vi "UHR-Fleezers Control (host) - 12.1_Jonathan.vi"() -> ()   [LabVIEW 2012] (continued)
            n2498 = VISA Write(VISA resource name=w4134, write buffer=w4133) -> (VISA resource name out=w4130:refnum<visa-resource-name>)  [unwired: 1 in, 2 out]
            n2499 = Concatenate Strings("cvolume" ("string"), "\r") -> (w4131:string)
            n2500 = VISA Write(VISA resource name=w4130, write buffer=w4131) -> (VISA resource name out=w4125:refnum<visa-resource-name>)  [unwired: 1 in, 2 out]
            n2501 = Concatenate Strings("wrun" ("string"), "\r") -> (w4126:string)
            n2502 = VISA Write(VISA resource name=w4125, write buffer=w4126) -> ()  [unwired: 1 in, 3 out]
          }
        }
      }
      event "Flip Green Filter": Value Change {
        n2503 = event-data() -> ()  [unwired: 7 out]
        n2504 = Not(x="Flip Green Filter") -> (.not. x?=w4144:bool)
        n2505 = local write "Flip Green Filter"(w4144) -> ()
        n2506 = flat-sequence {
          tunnel: w4152 -> [w4157]
          tunnel: w4151 -> [w4156]
          tunnel: [w4154] -> w4149
          tunnel: [w4153] -> w4148
          tunnel: [w4159] -> w4147
          tunnel: w4149 -> [w4159]
          tunnel: [w4158] -> w4146
          tunnel: w4148 -> [w4158]
          tunnel: w4147 -> [w4163]
          tunnel: w4146 -> [w4162]
          tunnel: [w4161] -> w4150
          frame #0 {
            n2507 = xnode "Read/Write Control"("FPGA VI Reference In"=w4157, "error in"=w4156, "Green Filter Flipper"=TRUE) -> ("FPGA VI Reference Out"=w4154:T20, "error out"=w4153:errorcluster)
          }
          frame #1 {
            n2508 = Wait (ms)(milliseconds to wait=u32 100) -> ()  [unwired: 1 out]
          }
          frame #2 {
            n2509 = xnode "Read/Write Control"("FPGA VI Reference In"=w4163, "error in"=w4162, "Green Filter Flipper"=FALSE) -> ("error out"=w4161:errorcluster)  [unwired: 1 out]
          }
        }
      }
      event "Pump 1 contents", "Pump 3 contents": Value Change {
        n2510 = event-data() -> ()  [unwired: 7 out]
        n2511 = local read "Pump 1 contents"() -> (→"Pump 1 cont disp":string)
        n2512 = local read "Pump 3 contents"() -> (→"Pump 3 cont disp":string)
      }
      event "Reset Trap Pos. FB": Value Change {
        n2513 = event-data() -> ()  [unwired: 7 out]
        n2514 = xnode "Read/Write Control"("FPGA VI Reference In"=w4169, "error in"=w4168, "Trap Pos. FB Reset"="Reset Trap Pos. FB") -> ()  [unwired: 2 out]
      }
      event "Rem fb disp offset": Value Change {
        n2515 = event-data() -> ()  [unwired: 7 out]
        n2516 = local write "Rem fb disp offset"(FALSE ("Rem fb disp offset")) -> ()
        n2517 = local read "Mean T1 Position (nm)"() -> (w4171:dbl)
        n2518 = local read "FB Trap Pos Offset"() -> (w4172:dbl)
        n2519 = Subtract(x=w4172, y=w4171) -> (x-y=w4170:dbl)
        n2520 = local write "FB Trap Pos Offset"(w4170) -> ()
      }
      event "Threshold (nm)": Value Change {
        n2521 = event-data() -> ()  [unwired: 7 out]
        n2522 = flat-sequence {
          tunnel: w4176 -> [w4184]
          tunnel: w4175 -> [w4183]
          tunnel: [w4177] -> w4174
          tunnel: w4174 -> [w4190]
          frame #0 {
            n2523 = xnode "Read/Write Control"("FPGA VI Reference In"=w4184, "error in"=w4183) -> ("FPGA VI Reference Out"=w4180:T20, "error out"=w4179:errorcluster, "FPGA TTrig Thresh"=w4181:i64)
            n2524 = local read "Threshold stored (nm)"() -> (w4189:dbl)
            n2525 = local read "Threshold (nm)"() -> (w4177:dbl)
            n2526 = local read "AOM X Cal (nm/MHz)"() -> (w4187:dbl)
            n2527 = Subtract(x=w4177, y=w4189) -> (x-y=w4188:dbl)
            n2528 = Divide(x=w4188, y=w4187) -> (x/y=w4185:dbl)
            n2529 = call "IR AOM freq to word.vi"("Frequency In (MHz)"=w4185) -> ("Frequency Word Out (double)"=w4186:dbl)
            n2530 = To Quad Integer(1:w4186) -> (0:w4182:i64)
            n2531 = Add(x=w4181, y=w4182) -> (x+y=w4178:i64)
            n2532 = xnode "Read/Write Control"("FPGA VI Reference In"=w4180, "error in"=w4179, "FPGA TTrig Thresh"=w4178) -> ()  [unwired: 2 out]
          }
          frame #1 {
            "Threshold stored (nm)" <- w4190
          }
        }
      }
      event "FB Trig Integrate": Value Change {
        n2533 = event-data() -> ()  [unwired: 7 out]
        n2534 = local read "FB Trig Integrate"() -> (w4192:u32)
        n2535 = xnode "Read/Write Control"("FPGA VI Reference In"=w4194, "error in"=w4193, "FB Trig Integrate"=w4192) -> ("error out"=w4191:errorcluster)  [unwired: 1 out]
      }
      event "11": Value Change {
        n2536 = event-data() -> ()  [unwired: 7 out]
        n2537 = local read "11"() -> (w4195:bool)
        n2538 = case shown="True" w4195 {
          frame False {
          }
          frame True {
            n2539 = local read "Messages"() -> (w4197:string)
            n2540 = call "Update messages.vi"("Message to add"="You kicked it up to 11!", "Old message string"=w4197) -> ("New message string"=w4198:string)
            n2541 = call <vilib>:"Beep.vi"() -> ()  [unwired: 12 in]
            n2542 = local write "Messages"(w4198) -> ()
          }
        }
      }
      event "Trap Pos. FB ON": Value Change {
        n2543 = event-data() -> ()  [unwired: 7 out]
        n2544 = xnode "Read/Write Control"("FPGA VI Reference In"=w4201, "error in"=w4200, "Force feedback"="Trap Pos. FB ON") -> ()  [unwired: 2 out]
      }
      event "Remove Action Offset": Value Change {
        n2545 = event-data() -> ()  [unwired: 7 out]
        n2546 = local write "Remove Action Offset"(FALSE ("Remove Action Offset")) -> ()
        n2547 = local read "Trap Pos. FB Mult Factor"() -> (w4206:i64)
        n2548 = local read "Trap Pos FB Action"() -> (w4204:i64)
        n2549 = local read "Trap Pos. FB Offset Factor"() -> (w4202:i64)
        n2550 = Multiply(x=w4206, y=w4204) -> (x*y=w4205:i64)
        n2551 = Add(x=w4205, y=w4202) -> (x+y=w4203:i64)
        n2552 = local write "Trap Pos. FB Offset Factor"(w4203) -> ()
        n2553 = xnode "Read/Write Control"("FPGA VI Reference In"=w4209, "error in"=w4208, "Trap Pos. FB Offset Factor"=w4203) -> ()  [unwired: 2 out]
      }
      event "Remove Unwinding Offset": Value Change {
        n2554 = event-data() -> ()  [unwired: 7 out]
        n2555 = local write "Remove Unwinding Offset"(FALSE ("Remove Action Offset")) -> ()
        n2556 = local read "Trap Pos. FB Mult Factor"() -> (w4221:i64)
        n2557 = local read "Trap Pos FB Action"() -> (w4219:i64)
        n2558 = local read "Trap Pos. FB Offset Factor"() -> (w4218:i64)
        n2559 = Multiply(x=w4221, y=w4219) -> (x*y=w4220:i64)
        n2560 = local read "Trap Pos. FB Mult Factor"() -> (w4217:i64)
        n2561 = Add(x=w4220, y=w4218) -> (x+y=w4211:i64)
        n2562 = Multiply(x=32768, y="factor") -> (x*y=w4214:dbl)
        n2563 = Multiply(x=w4214, y=w4217) -> (x*y=w4216:dbl)
        n2564 = Subtract(x=w4211, y=w4216) -> (x-y=w4215:dbl)
        n2565 = To Quad Integer(1:w4215) -> (0:w4210:i64)
        n2566 = xnode "Read/Write Control"("FPGA VI Reference In"=w4224, "error in"=w4223, "Trap Pos. FB Offset Factor"=w4210) -> ()  [unwired: 2 out]
        n2567 = local write "Trap Pos. FB Offset Factor"(w4210) -> ()
      }
      event "Trap Pos. FB Range", "Trap Pos. FB Gains", "Trap Pos. FB Mult Factor", "Trap Pos. FB Offset Factor", "Trap Pos FB Negate Action", "Trap Pos FB Monitor\nT1 or T2", "Differential FB?", "Negate Diff?": Value Change {
        n2568 = event-data() -> ()  [unwired: 7 out]
        n2569 = local read "Negate Diff?"() -> (w4225:bool)
        n2570 = xnode "Read/Write Control"("FPGA VI Reference In"=w4235, "error in"=w4234, "Trap Pos. FB Range"="Trap Pos. FB Range", "Trap Pos. FB Gains"="Trap Pos. FB Gains", "Trap Pos. FB Mult Factor"="Trap Pos. FB Mult Factor", "Trap Pos. FB Offset Factor"="Trap Pos. FB Offset Factor", "Trap Pos FB Negate Action"="Trap Pos FB Negate Action", "Trap Pos FB Monitor T1 or T2"="Trap Pos FB Monitor\nT1 or T2", "AI1 X Scale"="Trap Pos. AI1 X Pre-scale", "Negate Diff?"=w4225, "Diff FB Measurement?"="Differential FB?") -> ()  [unwired: 2 out]
      }
      event "Trap Pos FB SP", "Trap Pos FB SP 2", "Use SP 2": Value Change {
        n2571 = event-data() -> ()  [unwired: 7 out]
        n2572 = Select(t="Trap Pos FB SP 2", s="Use SP 2", f="Trap Pos FB SP") -> (s? t:f=w4236:fxp<+/-,16,1>)
        n2573 = xnode "Read/Write Control"("FPGA VI Reference In"=w4241, "error in"=w4240, "Trap Pos. FB SP"=w4236) -> ()  [unwired: 2 out]
      }
      event "Offset SP2 from SP1": Value Change {
        n2574 = event-data() -> ()  [unwired: 7 out]
        n2575 = local read "Trap Pos FB SP"() -> (w4244:fxp<+/-,16,1>)
        n2576 = Add(x=w4244, y="SP2 Offset") -> (x+y=w4242:fxp<+/-,16,1>)
        n2577 = property on="Trap Pos FB SP 2" class="DigNum (strict)"("Val(Sgnl)"=w4242) -> ()  [unwired: 2 in, 2 out]
        n2578 = local write "Offset SP2 from SP1"(FALSE ("Offset SP2 from SP1")) -> ()
      }
      event "Set Reading to\nSetpoint": Value Change {
        # "This is the actual PID input signal"
        n2579 = event-data() -> ()  [unwired: 7 out]
        n2580 = local write "Set Reading to\nSetpoint"(FALSE ("Set SP to Reading")) -> ()
        n2581 = xnode "Read/Write Control"("FPGA VI Reference In"=w4250, "error in"=w4249) -> ("FPGA VI Reference Out"=w4248:T20, "error out"=w4247:errorcluster, "Trap Pos FB Int-Norm Signal"=w4246:fxp<+/-,16,1>)
        n2582 = local read "Differential FB?"() -> (w4251:bool)
        n2583 = case shown="False" w4251 {
          tunnel: [w4256 w4263] -> w4253
          tunnel: w4246 -> [w4254 w4263]
          frame False {
            n2584 = local read "Trap Pos FB Monitor\nT1 or T2"() -> (w4259:bool)
            n2585 = local read "Trap X AI1 (DMA)"() -> (w4262:T14)
            n2586 = Unbundle By Name(w4262) -> ("Set 1"=w4261:fxp<+/-,16,1>, "Set 2"=w4260:fxp<+/-,16,1>)
            n2587 = Select(t=w4261, s=w4259, f=w4260) -> (s? t:f=w4258:fxp<+/-,16,1>)
            n2588 = Not(x="Set SP Using...") -> (.not. x?=w4255:bool)
            n2589 = Select(t=w4254, s=w4255, f=w4258) -> (s? t:f=w4256:fxp<+/-,16,1>)
          }
          frame True {
          }
        }
        n2590 = xnode "Read/Write Control"("FPGA VI Reference In"=w4248, "error in"=w4247, "Trap Pos. FB SP"=w4253) -> ()  [unwired: 2 out]
        n2591 = local write "Trap Pos FB SP"(w4253) -> ()
      }
      event "Trap Pos. FB Out Scale 2^n": Value Change {
        n2592 = event-data() -> ()  [unwired: 7 out]
        n2593 = Scale By Power Of 2(n="Trap Pos. FB Out Scale 2^n", x=ext 1.0) -> (x*2^n=w4264:ext)
        n2594 = property on="Trap Pos. FB Mult Factor" class="DigNum (strict)"("Val(Sgnl)"=w4264) -> ()  [unwired: 2 in, 2 out]
      }
      event "Trap Pos FB Int Count": Value Change {
        n2595 = event-data() -> ()  [unwired: 7 out]
        n2596 = xnode "Read/Write Control"("FPGA VI Reference In"=w4269, "error in"=w4268, "Trap Pos FB Int Count"="Trap Pos FB Int Count") -> ()  [unwired: 2 out]
      }
      event "Trap pos": Value Change {
        n2597 = event-data() -> ()  [unwired: 7 out]
        n2598 = case shown="True" "Trap pos" {
          frame False {
            n2599 = property on="Trap Delta Graph" class="WFGraph (strict)"("Visible"=TRUE) -> ()  [unwired: 2 in, 2 out]
            n2600 = property on="Saved trap pos" class="WFGraph (strict)"("Visible"=FALSE) -> ()  [unwired: 2 in, 2 out]
          }
          frame True {
            n2601 = property on="Saved trap pos" class="WFGraph (strict)"("Visible"=TRUE) -> ()  [unwired: 2 in, 2 out]
            n2602 = property on="Trap Delta Graph" class="WFGraph (strict)"("Visible"=FALSE) -> ()  [unwired: 2 in, 2 out]
          }
        }
      }
    }
    "error out 2" <- w3174
    n2603 = node-c288() -> ()  [unwired: 2 out]
  }
  n2604 = timed-loop "Oscillate Trap/AOM (fishing, debugging)" {
    tunnel: w8 -> [w4276]
    tunnel: [w4275] -> w102
    timing: w97 -> [_]
    timing-out: [_] -> w96
    stop <- w4275 stop-if-true
    n2605 = node-c288() -> ()  [unwired: 2 out]
    n2606 = event shown="[0] \"Oscillate Set 1\", \"Fish for Tether\": Value Change" {
      selector: _ -> [_ _ _]
      dyn-events: _ -> [_ _ _]
      timeout: _ -> [_ _ _]
      tunnel: w4276 -> [w4283 _ _]
      tunnel: [FALSE ("Stop All") _ w4872] -> w4275
      event "Oscillate Set 1", "Fish for Tether": Value Change {
        n2607 = event-data() -> ()  [unwired: 6 out]
        n2608 = local read "Oscillate Set 1"() -> (w4282:bool)
        n2609 = Or(x=w4282, y="Fish for Tether") -> (x .or. y?=w4280:bool)
        n2610 = case shown="True" w4280 {
          tunnel: w4283 -> [_ w4286]
          tunnel: "Fish for Tether" -> [_ w4285]
          frame False {
          }
          frame True {
            n2611 = case shown="True" w4285 {
              selector: w4285 -> [w4289 w4295]
              tunnel: [w4289 w4295] -> w4284
              frame False {
              }
              frame True {
                n2612 = local write "Scan axis 2"(TRUE) -> ()
                n2613 = local write "Tether"(FALSE ("Tether")) -> ()
                n2614 = local read "Flow ON during cal?"() -> (w4290:bool)
                n2615 = property on="Trap Delta (MHz)" class="DigNum (strict)"("Val(Sgnl)"="Furthest Delta (MHz)") -> ()  [unwired: 2 in, 2 out]
                n2616 = Or(x="Flow ON during \nfishing?", y=w4290) -> (x .or. y?=w4291:bool)
                n2617 = Wait (ms)(milliseconds to wait=u32 500) -> ()  [unwired: 1 out]
                n2618 = property on="Sample Channel\nFlow" class="Bool (strict)"("Val(Sgnl)"=w4291) -> ()  [unwired: 2 in, 2 out]
              }
            }
            n2619 = node-c288() -> (w4288:T22)  [unwired: 4 out]
            n2620 = timed-loop "Oscillate AOD" {
              timing: w4288 -> [_]
              timing-out: [_] -> w4287
              tunnel: w4286 -> [w4305]
              tunnel: w4284 -> [w4298]
              i -> [w4307]
              stop <- w4304 stop-if-true
              n2621 = node-c288() -> (w4306:i64)  [unwired: 1 out]
              n2622 = flat-sequence {
                tunnel: w4307 -> [w4334]
                tunnel: w4306 -> [w4333]
                tunnel: w4305 -> [w4312]
                tunnel: w4298 -> [w4315]
                tunnel: [w4315] -> w4303
                tunnel: [w4314] -> w4302
                tunnel: [w4311] -> w4301
                tunnel: [w4308] -> w4299
                tunnel: w4303 -> [w4370]
                tunnel: w4302 -> [w4368]
                tunnel: w4301 -> [w4367]
                tunnel: [w4366] -> w4300
                tunnel: w4299 -> [w4365]
                tunnel: [w4442] -> w4304
                tunnel: w4300 -> [w4441]
                frame #0 {
                  n2623 = Divide(x=w4333, y=i64 1000) -> (x/y=w4328:dbl)
                  n2624 = Multiply(x=w4328, y=w4334) -> (x*y=w4330:dbl)
                  n2625 = local read "BD 1 Frequency 2 (MHz)"() -> (w4313:dbl)
                  n2626 = Multiply(x="Osc. freq. (Hz)", y=6.283185307179586) -> (x*y=w4331:dbl)
                  n2627 = Multiply(x=w4331, y=w4330) -> (x*y=w4310:dbl)
                  n2628 = local read "BD 1 Frequency 1 (MHz)"() -> (w4318:dbl)
                  n2629 = local read "BD 2 Frequency 1 (MHz)"() -> (w4317:dbl)
                  n2630 = case shown="True" w4315 {
                    tunnel: w4310 -> [w4340 w4345]
                    tunnel: w4318 -> [_ w4356]
                    tunnel: w4313 -> [_ w4357]
                    tunnel: [w4337 w4351] -> w4316
                    tunnel: [FALSE w4348] -> w4311
                    tunnel: [0.0 w4341] -> w4308
                    frame False {
                      n2631 = Sine(x=w4340) -> (sin(x)=w4338:dbl)
                      n2632 = Multiply(x=w4338, y="Osc. amp. (MHz)") -> (x*y=w4337:dbl)
                    }
                    frame True {
                      n2633 = Cosine(x=w4345) -> (cos(x)=w4360:dbl)
                      n2634 = Subtract(x=w4357, y=w4356) -> (x-y=w4355:dbl)
                      n2635 = Decrement(x=w4360) -> (x-1=w4359:dbl)
                      n2636 = Subtract(x=w4355, y="Closest Delta (MHz)") -> (x-y=w4352:dbl)
                      n2637 = Divide(x=w4359, y=-2.0) -> (x/y=w4353:dbl)
                      n2638 = Multiply(x=w4353, y=w4352) -> (x*y=w4351:dbl)
                      n2639 = local read "Vec Mean of T1 T2"() -> (w4347:dbl[])
                      n2640 = Greater?(x=w4347, y="Stop F (pN)") -> (0:w4349:bool[])
                      n2641 = Or Array Elements(Boolean array=w4349) -> (logical OR=w4348:bool)
                      n2642 = Divide(x=w4345, y=6.283185307179586) -> (x/y=w4344:dbl)
                      n2643 = Round Toward +Infinity(x=w4344) -> (ceil(x): smallest int >= x=w4341:dbl)
                      "Attempts" <- w4341
                      n2644 = Greater?(x=w4341, y="Attempt Limit") -> (0:w4343:bool)
                      n2645 = case shown="True" w4343 {
                        frame False {
                        }
                        frame True {
                          n2646 = local write "Fish for Tether"(FALSE ("Fish for Tether")) -> ()
                          n2647 = call <vilib>:"Beep.vi"() -> ()  [unwired: 3 in, 9 out]
                          n2648 = local read "Messages"() -> (w4362:string)
                          n2649 = call "Update messages.vi"("Message to add"="Tether fishing timeout." ("Messages"), "Old message string"=w4362) -> ("New message string"=→"Messages":string)
                        }
                      }
                    }
                  }
                  n2650 = Select(t=w4318, s="Scan axis 2", f=w4317) -> (s? t:f=w4321:dbl)
                  n2651 = Add(x=w4316, y=w4321) -> (x+y=w4314:dbl)
                  n2652 = Select(t=w4314, s="Scan axis 2", f=w4318) -> (s? t:f=w4324:dbl)
                  n2653 = Select(t=w4317, s="Scan axis 2", f=w4314) -> (s? t:f=w4323:dbl)
                  n2654 = local read "Y RF Frequency Limits (MHz)"() -> (w4319:T17)
                  n2655 = local read "X RF Frequency Limits (MHz)"() -> (w4320:T17)
                  n2656 = local read "BD 1 Frequency 3 (MHz)"() -> (w4327:dbl)
                  n2657 = local read "BD 2 Frequency 2 (MHz)"() -> (w4326:dbl)
                  n2658 = local read "BD 2 Frequency 3 (MHz)"() -> (w4325:dbl)
                  n2659 = call "set RF board frequency - interlace.vi"("Board 2 Frequency Limits"=w4319, "Board 1 Frequency Limits"=w4320, "FPGA VI Reference In"=w4312, "Board 2 Frequency 3 (MHz)"=w4325, "Board 1 Frequency 3 (MHz)"=w4327, "Board 2 Frequency 2 (MHz)"=w4326, "Board 2 Frequency 1 (MHz)"=w4323, "Board 1 Frequency 2 (MHz)"=w4313, "Board 1 Frequency 1  (MHz)"=w4324) -> ()  [unwired: 1 in, 2 out]
                }
                frame #1 {
                  n2660 = And(x=w4370, y=w4367) -> (x .and. y?=w4369:bool)
                  n2661 = case "Only if were fishing and now formed tether" shown="False" w4369 {
                    tunnel: w4368 -> [w4372 w4387]
                    tunnel: [w4371 w4386] -> w4366
                    tunnel: w4365 -> [_ w4382]
                    frame False {
                      n2662 = local read "Fish for Tether"() -> (w4371:bool)
                      n2663 = case shown="False" w4371 {
                        tunnel: w4372 -> [w4373 _]
                        frame False {
                          n2664 = property on="BD 1 Frequency 1 (MHz)" class="DigNum (strict)"("Val(Sgnl)"=w4373) -> ()  [unwired: 2 in, 2 out]
                        }
                        frame True {
                        }
                      }
                    }
                    frame True {
                      w4386 = FALSE ("Fish for Tether")
                      n2665 = call <vilib>:"Beep.vi"() -> ()  [unwired: 3 in, 9 out]
                      n2666 = Number To Decimal String(number=w4382, width (-)=i16 1) -> (decimal integer string=w4380:string)
                      n2667 = Concatenate Strings("Formed tether in ", w4380, " attempt(s)." ("string")) -> (w4377:string)
                      n2668 = local read "Messages"() -> (w4384:string)
                      n2669 = local write "Fish for Tether"(w4386) -> ()
                      n2670 = call "Update messages.vi"("Message to add"=w4377, "Old message string"=w4384) -> ("New message string"=w4383:string)
                      n2671 = local write "Messages"(w4383) -> ()
                      n2672 = Get Date/Time In Seconds() -> (seconds since 1Jan1904=→"Time tether formed":timestamp)
                      n2673 = local read "Flow ON during cal?"() -> (w4374:bool)
                      n2674 = property on="Sample Channel\nFlow" class="Bool (strict)"("Val(Sgnl)"=w4374) -> (error out=w4375:errorcluster)  [unwired: 2 in, 1 out]
                      n2675 = case shown="\"2\", \"3\", \"4\", \"5\", \"6\"" "Then..." {
                        selector: "Then..." -> [_ w4390]
                        tunnel: w4387 -> [w4389 _]
                        tunnel: w4375 -> [_ _]
                        frame "1", Default {
                          n2676 = property on="BD 1 Frequency 1 (MHz)" class="DigNum (strict)"("Val(Sgnl)"=w4389) -> ()  [unwired: 2 in, 2 out]
                        }
                        frame "2", "3", "4", "5", "6" {
                          n2677 = flat-sequence {
                            tunnel: w4390 -> [w4392]
                            frame #0 {
                              n2678 = property on="Trap Delta (MHz)" class="DigNum (strict)"("Val(Sgnl)"="Move to Delta 1 (MHz)") -> ()  [unwired: 2 in, 2 out]
                            }
                            frame #1 {
                              n2679 = case shown="\"5\", \"6\"" w4392 {
                                selector: w4392 -> [w4395 w4405 _]
                                frame "3", "4" {
                                n2680 = flat-sequence {
                                tunnel: w4395 -> [w4396]
                                tunnel: [w4396] -> w4393
                                tunnel: [w4398] -> w4394
                                tunnel: w4393 -> [w4398]
                                tunnel: w4394 -> [w4402]
                                frame #0 {
                                n2681 = property on="Green Laser ON/Interlacing" class="Bool (strict)"("Val(Sgnl)"=TRUE ("Value (Signaling)")) -> ()  [unwired: 2 in, 2 out]
                                }
                                frame #1 {
                                n2682 = Multiply(x="Wait Before Save (s)", y=u32 1000 ("x")) -> (x*y=w4400:u32)
                                n2683 = Wait (ms)(milliseconds to wait=w4400) -> ()  [unwired: 1 out]
                                }
                                frame #2 {
                                n2684 = property on="Start Saving" class="Bool (strict)"("Value"=TRUE ("Start Saving")) -> ()  [unwired: 2 in, 2 out]
                                n2685 = case shown="\"4\"" w4402 {
                                frame Default {
                                }
                                frame "4" {
                                n2686 = property on="Fl. Triggered..." class="Bool (strict)"("Val(Sgnl)"=TRUE ("Value (Signaling)")) -> ()  [unwired: 2 in, 2 out]
                                }
                                }
                                }
                                }
                                }
                                frame "5", "6" {
                                n2687 = stacked-sequence {
                                tunnel: w4405 -> [_ _ _ _ _ _ w4417]
                                frame #0 {
                                n2688 = Replace Array Subset(array=u32[] [0] ("Index Values"), new element="Raster Set Upon Tether", index=0) -> (w4406:u32[])
                                n2689 = property on="Saved AOD Raster Scan Parameter Sets" class="Arr (strict)"("Index Values"=w4406) -> ()  [unwired: 2 in, 2 out]
                                }
                                frame #1 {
                                n2690 = Wait (ms)(milliseconds to wait=u32 500) -> ()  [unwired: 1 out]
                                }
                                frame #2 {
                                n2691 = property on="Load parameters" class="Bool (strict)"("Val(Sgnl)"=TRUE ("Value (Signaling)")) -> ()  [unwired: 2 in, 2 out]
                                n2692 = case shown="True" "Green ON During Raster" {
                                frame False {
                                }
                                frame True {
                                n2693 = property on="Green Laser ON/Interlacing" class="Bool (strict)"("Val(Sgnl)"=TRUE ("Value (Signaling)")) -> ()  [unwired: 2 in, 2 out]
                                }
                                }
                                }
                                frame #3 {
                                n2694 = Wait (ms)(milliseconds to wait=u32 500) -> ()  [unwired: 1 out]
                                }
                                frame #4 {
                                n2695 = property on="Trap Raster Scan" class="Bool (strict)"("Val(Sgnl)"=TRUE ("Value (Signaling)")) -> ()  [unwired: 2 in, 2 out]
                                }
                                frame #5 {
                                n2696 = Wait (ms)(milliseconds to wait=u32 2000) -> ()  [unwired: 1 out]
                                }
                                frame #6 {
                                n2697 = flat-sequence {
                                tunnel: w4417 -> [w4424]
                                frame #0 {
                                n2698 = while {
                                stop <- w4420 stop-if-true
                                n2699 = local read "Raster Scanning..."() -> (w4419:bool)
                                n2700 = local read "Saving..."() -> (w4422:bool)
                                n2701 = Wait (ms)(milliseconds to wait=u32 100) -> ()  [unwired: 1 out]
                                n2702 = Not(x=w4422) -> (.not. x?=w4421:bool)
                                n2703 = Not(x=w4419) -> (.not. x?=w4418:bool)
                                n2704 = And(x=w4421, y=w4418) -> (x .and. y?=w4420:bool)
                                }
                                }
                                frame #1 {
                                n2705 = local read "Tether"() -> (w4425:bool)
                                n2706 = case shown="True" w4425 {
                                tunnel: w4424 -> [_ w4427]
                                frame False {
                                n2707 = property on="Fish for Tether" class="Bool (strict)"("Val(Sgnl)"="Fish again after \nraster break?") -> ()  [unwired: 2 in, 2 out]
                                }
                                frame True {
                                n2708 = stacked-sequence {
                                tunnel: w4427 -> [_ w4431 _ _]
                                frame #0 {
                                n2709 = property on="Trap Delta (MHz)" class="DigNum (strict)"("Val(Sgnl)"="Move to Delta 2 (MHz)") -> ()  [unwired: 2 in, 2 out]
                                n2710 = case shown="True" "Flow ON after\ntether testing?" {
                                frame False {
                                }
                                frame True {
                                n2711 = property on="Sample Channel\nFlow" class="Bool (strict)"("Val(Sgnl)"=TRUE ("Value (Signaling)")) -> ()  [unwired: 2 in, 2 out]
                                }
                                }
                                }
                                frame #1 {
                                n2712 = flat-sequence {
                                tunnel: w4431 -> [w4433]
                                frame #0 {
                                n2713 = Wait (ms)(milliseconds to wait=u32 500) -> ()  [unwired: 1 out]
                                }
                                frame #1 {
                                n2714 = case shown="\"6\"" w4433 {
                                frame Default {
                                }
                                frame "6" {
                                n2715 = property on="Green Laser ON/Interlacing" class="Bool (strict)"("Val(Sgnl)"=TRUE ("Green Laser ON/Interlacing")) -> ()  [unwired: 2 in, 2 out]
                                }
                                }
                                }
                                frame #2 {
                                n2716 = Wait (ms)(milliseconds to wait=u32 500) -> ()  [unwired: 1 out]
                                }
                                frame #3 {
                                n2717 = local write "Start Saving"("Save at end (5, 6)") -> ()
                                }
                                }
                                }
                                frame #2 {
                                n2718 = local read "Bead Sep. Int. Time (s)"() -> (w4439:dbl)
                                n2719 = Multiply(x=w4439, y=1000.0) -> (x*y=w4438:dbl)
                                n2720 = Wait (ms)(milliseconds to wait=w4438) -> ()  [unwired: 1 out]
                                }
                                frame #3 {
                                n2721 = property on="Remove Offset" class="Bool (strict)"("Val(Sgnl)"=TRUE ("Value (Signaling)")) -> ()  [unwired: 2 in, 2 out]
                                }
                                }
                                }
                                }
                                }
                                }
                                }
                                }
                                }
                                frame "2", Default {
                                }
                              }
                            }
                          }
                        }
                      }
                      "Tether" <- "Tether Alarm?"
                    }
                  }
                }
                frame #2 {
                  n2722 = local read "Oscillate Set 1"() -> (w4446:bool)
                  n2723 = local read "Stop All"() -> (w4444:bool)
                  n2724 = Or(x=w4446, y=w4441) -> (x .or. y?=w4443:bool)
                  n2725 = Not(x=w4443) -> (.not. x?=w4445:bool)
                  n2726 = Compound Arithmetic op=OR(w4444, w4445) -> (w4442:bool)
                }
              }
              n2727 = node-c288() -> ()  [unwired: 2 out]
            }
            n2728 = node-c288(w4287) -> ()  [unwired: 1 out]
          }
        }
      }
      event "Fl. Triggered...": Value Change {
        n2729 = event-data() -> ()  [unwired: 7 out]
        n2730 = case shown="True" "Fl. Triggered..." {
          frame False {
          }
          frame True {
            n2731 = node-c288() -> (w4457:T22)  [unwired: 4 out]
            n2732 = timed-loop {
              timing: w4457 -> [_]
              timing-out: [_] -> w4456
              tunnel: "Action" -> [w4465]
              shift-right: [w4462] -> _
              shift-left: u8 255 -> [w4464]
              shift-right: [w4459] -> _
              shift-left: 255 -> [w4461]
              stop <- w4458 stop-if-true
              # "Reset confocal spot"
              n2733 = node-c288() -> ()  [unwired: 2 out]
              n2734 = flat-sequence {
                tunnel: w4465 -> [w4485]
                tunnel: w4464 -> [w4484]
                tunnel: [w4483] -> w4463
                tunnel: w4461 -> [w4470]
                tunnel: [w4469] -> w4460
                tunnel: [w4864] -> w4458
                tunnel: w4463 -> [w4863]
                tunnel: [w4863] -> w4462
                tunnel: [w4862] -> w4459
                tunnel: w4460 -> [w4862]
                frame #0 {
                  n2735 = local read "Delta Fl. 2"() -> (w4482:dbl)
                  n2736 = local read "Delta Fl. 1"() -> (w4477:dbl)
                  n2737 = Multiply(x="Fl. Delta Thresh. (kHz)", y=1000.0) -> (x*y=w4472:dbl)
                  n2738 = Select(t=w4477, s="APD to Watch", f=w4482) -> (s? t:f=w4473:dbl)
                  n2739 = Greater?(x=w4473, y=w4472) -> (0:w4478:bool)
                  n2740 = Or(x="Force Yank", y=w4478) -> (x .or. y?=w4476:bool)
                  n2741 = And(x=w4476, y="Yank when?") -> (x .and. y?=w4474:bool)
                  n2742 = case shown="False" w4474 {
                    tunnel: w4485 -> [w4488 w4689]
                    tunnel: w4484 -> [w4490 w4685]
                    tunnel: [w4490 w4683] -> w4483
                    tunnel: w4473 -> [w4496 _]
                    tunnel: w4472 -> [w4495 _]
                    tunnel: "Force Yank" -> [w4493 _]
                    tunnel: w4470 -> [w4492 w4682]
                    tunnel: [w4491 w4682] -> w4469
                    frame False {
                      n2743 = Negate(x=w4495) -> (-x=w4487:dbl)
                      n2744 = local write "Fl. High"(TRUE ("Fl. High")) -> ()
                      n2745 = Less?(x=w4496, y=w4487) -> (x < y?=w4494:bool)
                      n2746 = Or(x=w4493, y=w4494) -> (x .or. y?=w4489:bool)
                      n2747 = case shown="True" w4489 {
                        tunnel: w4492 -> [w4497 w4507]
                        tunnel: [w4497 w4506] -> w4491
                        tunnel: w4488 -> [_ w4505]
                        frame False {
                        }
                        frame True {
                          n2748 = flat-sequence {
                            tunnel: w4507 -> [w4513]
                            tunnel: w4505 -> [w4510]
                            tunnel: [w4512] -> w4504
                            tunnel: [w4511] -> w4503
                            tunnel: [w4510] -> w4502
                            tunnel: w4501 -> [w4509]
                            tunnel: [w4509] -> w4500
                            tunnel: w4499 -> [w4508]
                            tunnel: [w4508] -> w4498
                            tunnel: [w4584] -> w4506
                            tunnel: w4504 -> [w4584]
                            tunnel: w4503 -> [w4583]
                            tunnel: w4502 -> [w4582]
                            tunnel: w4500 -> [w4581]
                            tunnel: w4498 -> [w4580]
                            frame #0 {
                              n2749 = call <vilib>:"Beep.vi"() -> ()  [unwired: 12 in]
                              n2750 = local write "Waiting"(FALSE ("Waiting")) -> ()
                              n2751 = Increment(x=w4513) -> (x+1=w4512:i32)
                              n2752 = case shown="\"Yank\"" w4510 {
                                tunnel: w4512 -> [_ w4518 _]
                                frame "Alarm", Default {
                                }
                                frame "Yank" {
                                n2753 = flat-sequence {
                                tunnel: w4518 -> [w4521]
                                tunnel: [w4520] -> w4517
                                tunnel: [w4519] -> w4516
                                tunnel: w4517 -> [w4531]
                                tunnel: w4516 -> [w4532]
                                frame #0 {
                                n2754 = local read "Yank Delay (s)"() -> (w4524:dbl)
                                n2755 = local read "N Array El"() -> (w4519:u8)
                                n2756 = Quotient & Remainder(x=w4521, y=w4519) -> (x-y*floor(x/y)=w4520:i32)  [unwired: 1 out]
                                n2757 = Multiply(x=w4524, y=1000.0) -> (x*y=w4522:dbl)
                                n2758 = Wait (ms)(milliseconds to wait=w4522) -> ()  [unwired: 1 out]
                                }
                                frame #1 {
                                n2759 = local read "Yank to which?"() -> (w4526:bool)
                                n2760 = local read "Random Choice"() -> (w4536:bool)
                                n2761 = local read "Yank to Trap Delta (MHz)"() -> (w4529:dbl[])
                                n2762 = local read "Yank to SP"() -> (w4530:dbl[])
                                n2763 = Random Number (0-1)() -> (number: 0 to 1=w4535:dbl)
                                n2764 = Multiply(x=w4532, y=w4535) -> (x*y=w4534:dbl)
                                n2765 = Round Toward -Infinity(1:w4534) -> (0:w4533:dbl)
                                n2766 = Select(t=w4533, s=w4536, f=w4531) -> (s? t:f=w4527:dbl)
                                n2767 = Select(t=w4529, s=w4526, f=w4530) -> (s? t:f=w4528:dbl[])
                                n2768 = Index Array(array=w4528, index=w4527) -> (element=w4525:dbl)
                                n2769 = case shown="True" w4526 {
                                tunnel: w4525 -> [w4537 w4564]
                                frame False {
                                n2770 = flat-sequence {
                                tunnel: w4537 -> [w4538]
                                frame #0 {
                                n2771 = property on="Trap Pos FB SP" class="DigNum (strict)"("Val(Sgnl)"=w4538) -> ()  [unwired: 2 in, 2 out]
                                }
                                frame #1 {
                                n2772 = Wait (ms)(milliseconds to wait=u32 700) -> ()  [unwired: 1 out]
                                }
                                frame #2 {
                                n2773 = local read "Action (%)"() -> (w4543:dbl)
                                n2774 = Absolute Value(x=w4543) -> (abs(x)=w4542:dbl)
                                n2775 = Greater?(x=w4542, y=70.0) -> (0:w4540:bool)
                                n2776 = property on="Remove Action Offset" class="Bool (strict)"("Val(Sgnl)"=w4540) -> ()  [unwired: 2 in, 2 out]
                                }
                                frame #3 {
                                n2777 = for {
                                N: 4 -> [_]
                                n2778 = flat-sequence {
                                frame #0 {
                                n2779 = Wait (ms)(milliseconds to wait=u32 500) -> ()  [unwired: 1 out]
                                }
                                frame #1 {
                                n2780 = local read "Action (%)"() -> (w4549:dbl)
                                n2781 = Absolute Value(x=w4549) -> (abs(x)=w4548:dbl)
                                n2782 = Greater?(x=w4548, y=70.0) -> (0:w4546:bool)
                                n2783 = property on="Remove Action Offset" class="Bool (strict)"("Val(Sgnl)"=w4546) -> ()  [unwired: 2 in, 2 out]
                                }
                                }
                                }
                                }
                                frame #4 {
                                n2784 = Wait (ms)(milliseconds to wait=u32 500) -> ()  [unwired: 1 out]
                                }
                                frame #5 {
                                n2785 = local read "Mean"() -> (w4557:dbl)
                                n2786 = Greater?(x=w4557, y=11.0) -> (0:w4551:bool)
                                n2787 = Not(x=w4551) -> (.not. x?=w4552:bool)
                                n2788 = And(x=w4552, y="Shift confocal") -> (x .and. y?=w4554:bool)
                                n2789 = And(x=w4551, y="Shift confocal") -> (x .and. y?=w4555:bool)
                                n2790 = case shown="True" w4555 {
                                frame False {
                                }
                                frame True {
                                n2791 = local read "Confocal Y 2 (V)"() -> (w4561:dbl)
                                n2792 = local read "Confocal X 2 (V)"() -> (w4560:dbl)
                                n2793 = property on="AO1" class="Slide (strict)"("Val(Sgnl)"=w4561) -> ()  [unwired: 2 in, 2 out]
                                n2794 = property on="AO2" class="Slide (strict)"("Val(Sgnl)"=w4560) -> ()  [unwired: 2 in, 2 out]
                                }
                                }
                                n2795 = case shown="True" w4554 {
                                frame False {
                                }
                                frame True {
                                n2796 = local read "Confocal Y 1 (V)"() -> (w4559:dbl)
                                n2797 = local read "Confocal X 1 (V)"() -> (w4558:dbl)
                                n2798 = property on="AO1" class="Slide (strict)"("Val(Sgnl)"=w4559) -> ()  [unwired: 2 in, 2 out]
                                n2799 = property on="AO2" class="Slide (strict)"("Val(Sgnl)"=w4558) -> ()  [unwired: 2 in, 2 out]
                                }
                                }
                                }
                                frame #6 {
                                n2800 = Wait (ms)(milliseconds to wait=u32 1500) -> ()  [unwired: 1 out]
                                }
                                frame #7 {
                                n2801 = property on="Rem fb disp offset" class="Bool (strict)"("Val(Sgnl)"=TRUE ("Value (Signaling)")) -> ()  [unwired: 2 in, 2 out]
                                }
                                }
                                }
                                frame True {
                                n2802 = flat-sequence {
                                tunnel: w4564 -> [w4565]
                                frame #0 {
                                n2803 = property on="Trap Delta (MHz)" class="DigNum (strict)"("Val(Sgnl)"=w4565) -> ()  [unwired: 2 in, 2 out]
                                }
                                frame #1 {
                                n2804 = Wait (ms)(milliseconds to wait=u32 500) -> ()  [unwired: 1 out]
                                }
                                frame #2 {
                                n2805 = local read "Shift confocal"() -> (w4571:bool)
                                n2806 = local read "Mean"() -> (w4573:dbl)
                                n2807 = Greater?(x=w4573, y=11.0) -> (0:w4570:bool)
                                n2808 = Not(x=w4570) -> (.not. x?=w4569:bool)
                                n2809 = And(x=w4569, y=w4571) -> (x .and. y?=w4567:bool)
                                n2810 = And(x=w4570, y=w4571) -> (x .and. y?=w4568:bool)
                                n2811 = case shown="True" w4568 {
                                frame False {
                                }
                                frame True {
                                n2812 = local read "Confocal Y 2 (V)"() -> (w4577:dbl)
                                n2813 = local read "Confocal X 2 (V)"() -> (w4576:dbl)
                                n2814 = property on="AO2" class="Slide (strict)"("Val(Sgnl)"=w4576) -> ()  [unwired: 2 in, 2 out]
                                n2815 = property on="AO1" class="Slide (strict)"("Val(Sgnl)"=w4577) -> ()  [unwired: 2 in, 2 out]
                                }
                                }
                                n2816 = case shown="True" w4567 {
                                frame False {
                                }
                                frame True {
                                n2817 = local read "Confocal X 1 (V)"() -> (w4574:dbl)
                                n2818 = local read "Confocal Y 1 (V)"() -> (w4575:dbl)
                                n2819 = property on="AO2" class="Slide (strict)"("Val(Sgnl)"=w4574) -> ()  [unwired: 2 in, 2 out]
                                n2820 = property on="AO1" class="Slide (strict)"("Val(Sgnl)"=w4575) -> ()  [unwired: 2 in, 2 out]
                                }
                                }
                                }
                                }
                                }
                                }
                                }
                                }
                                }
                                frame "Image" {
                                n2821 = property on="Confocal Image" class="Bool (strict)"("Val(Sgnl)"=TRUE ("Value (Signaling)")) -> ()  [unwired: 2 in, 2 out]
                                }
                              }
                              n2822 = local write "Fl. High"(FALSE ("Fl. High")) -> ()
                              n2823 = local read "Time (s)"() -> (w4511:dbl)
                            }
                            frame #1 {
                              n2824 = case shown="True" "Auto F Reset" {
                                tunnel: w4583 -> [_ w4588]
                                tunnel: w4582 -> [_ w4587]
                                tunnel: w4581 -> [_ w4586]
                                tunnel: w4580 -> [_ w4585]
                                frame False {
                                }
                                frame True {
                                n2825 = node-c288() -> (w4590:T22)  [unwired: 4 in]
                                n2826 = timed-loop {
                                timing: w4590 -> [_]
                                timing-out: [_] -> w4589
                                tunnel: w4588 -> [w4595]
                                tunnel: w4587 -> [w4594]
                                tunnel: w4586 -> [w4593]
                                tunnel: w4585 -> [w4592]
                                stop <- w4591 stop-if-true
                                n2827 = node-c288() -> ()  [unwired: 1 in, 1 out]
                                n2828 = local read "Fl. Delta Thresh. (kHz)"() -> (w4604:dbl)
                                n2829 = local read "APD to Watch"() -> (w4605:bool)
                                n2830 = local read "Delta Fl. 1"() -> (w4606:dbl)
                                n2831 = local read "Delta Fl. 2"() -> (w4607:dbl)
                                n2832 = local read "Fl. Triggered..."() -> (w4598:bool)
                                n2833 = local read "Stop All"() -> (w4599:bool)
                                n2834 = local read "Reset Force"() -> (w4597:bool)
                                n2835 = Multiply(x=w4604, y=1000.0) -> (x*y=w4602:dbl)
                                n2836 = Not(x=w4598) -> (.not. x?=w4596:bool)
                                n2837 = Select(t=w4606, s=w4605, f=w4607) -> (s? t:f=w4601:dbl)
                                n2838 = Greater?(x=w4601, y=w4602) -> (0:w4600:bool)
                                n2839 = Compound Arithmetic op=OR(w4600, w4599, w4596, w4597) -> (w4591:bool)
                                n2840 = case shown="True" w4591 {
                                tunnel: w4595 -> [_ w4611]
                                tunnel: w4594 -> [_ w4615]
                                tunnel: w4593 -> [_ w4614]
                                tunnel: w4592 -> [_ w4613]
                                frame False {
                                }
                                frame True {
                                n2841 = case shown="\"Yank\"" w4615 {
                                tunnel: w4614 -> [_ w4625]
                                tunnel: w4613 -> [_ w4623]
                                frame "Image", Default {
                                }
                                frame "Yank" {
                                n2842 = flat-sequence {
                                tunnel: [w4628] -> w4626
                                tunnel: w4625 -> [w4628]
                                tunnel: [w4627] -> w4624
                                tunnel: w4623 -> [w4627]
                                tunnel: w4626 -> [w4634]
                                tunnel: w4624 -> [w4632]
                                frame #0 {
                                n2843 = local read "Yank Delay (s)"() -> (w4631:dbl)
                                n2844 = Multiply(x=w4631, y=1000.0) -> (x*y=w4629:dbl)
                                n2845 = Wait (ms)(milliseconds to wait=w4629) -> ()  [unwired: 1 out]
                                }
                                frame #1 {
                                n2846 = local read "Yank to which?"() -> (w4633:bool)
                                n2847 = case shown="False" w4633 {
                                tunnel: w4634 -> [_ w4662]
                                tunnel: w4632 -> [w4635 _]
                                frame False {
                                n2848 = flat-sequence {
                                tunnel: w4635 -> [w4636]
                                frame #0 {
                                n2849 = property on="Trap Pos FB SP" class="DigNum (strict)"("Val(Sgnl)"=w4636) -> ()  [unwired: 2 in, 2 out]
                                }
                                frame #1 {
                                n2850 = Wait (ms)(milliseconds to wait=u32 700) -> ()  [unwired: 1 out]
                                }
                                frame #2 {
                                n2851 = local read "Action (%)"() -> (w4641:dbl)
                                n2852 = Absolute Value(x=w4641) -> (abs(x)=w4640:dbl)
                                n2853 = Greater?(x=w4640, y=70.0) -> (0:w4638:bool)
                                n2854 = property on="Remove Action Offset" class="Bool (strict)"("Val(Sgnl)"=w4638) -> ()  [unwired: 2 in, 2 out]
                                }
                                frame #3 {
                                n2855 = for {
                                N: 4 -> [_]
                                n2856 = flat-sequence {
                                frame #0 {
                                n2857 = Wait (ms)(milliseconds to wait=u32 500) -> ()  [unwired: 1 out]
                                }
                                frame #1 {
                                n2858 = local read "Action (%)"() -> (w4647:dbl)
                                n2859 = Absolute Value(x=w4647) -> (abs(x)=w4646:dbl)
                                n2860 = Greater?(x=w4646, y=70.0) -> (0:w4644:bool)
                                n2861 = property on="Remove Action Offset" class="Bool (strict)"("Val(Sgnl)"=w4644) -> ()  [unwired: 2 in, 2 out]
                                }
                                }
                                }
                                }
                                frame #4 {
                                n2862 = Wait (ms)(milliseconds to wait=u32 500) -> ()  [unwired: 1 out]
                                }
                                frame #5 {
                                n2863 = local read "Shift confocal"() -> (w4652:bool)
                                n2864 = local read "Mean"() -> (w4655:dbl)
                                n2865 = Greater?(x=w4655, y=11.0) -> (0:w4651:bool)
                                n2866 = Not(x=w4651) -> (.not. x?=w4650:bool)
                                n2867 = And(x=w4651, y=w4652) -> (x .and. y?=w4653:bool)
                                n2868 = And(x=w4650, y=w4652) -> (x .and. y?=w4649:bool)
                                n2869 = case shown="True" w4653 {
                                frame False {
                                }
                                frame True {
                                n2870 = local read "Confocal X 2 (V)"() -> (w4658:dbl)
                                n2871 = local read "Confocal Y 2 (V)"() -> (w4659:dbl)
                                n2872 = property on="AO2" class="Slide (strict)"("Val(Sgnl)"=w4658) -> ()  [unwired: 2 in, 2 out]
                                n2873 = property on="AO1" class="Slide (strict)"("Val(Sgnl)"=w4659) -> ()  [unwired: 2 in, 2 out]
                                }
                                }
                                n2874 = case shown="True" w4649 {
                                frame False {
                                }
                                frame True {
                                n2875 = local read "Confocal Y 1 (V)"() -> (w4657:dbl)
                                n2876 = local read "Confocal X 1 (V)"() -> (w4656:dbl)
                                n2877 = property on="AO1" class="Slide (strict)"("Val(Sgnl)"=w4657) -> ()  [unwired: 2 in, 2 out]
                                n2878 = property on="AO2" class="Slide (strict)"("Val(Sgnl)"=w4656) -> ()  [unwired: 2 in, 2 out]
                                }
                                }
                                }
                                frame #6 {
                                n2879 = Wait (ms)(milliseconds to wait=u32 1500) -> ()  [unwired: 1 out]
                                }
                                frame #7 {
